vi "Save Model Digest.vi"(6 "Model group name":string="Summary", 7 "Group name":string="Summary", 8 "error in (no error)":errorcluster, 9 "Input onfiguration":T1={"Input File Path"=path "", "from scan..."=0, "...to scan"=0, "Lead resistance"=0.0, "Correct conductance "=FALSE, "Model parameters gap 1"={"Delta 1"=0.0, "Delta 2"=0.0, "Gama"=0.0, "Z"=0.0, "P"=0.0, "T"=0.0, "Integration range"=0.0, "Resolution"=0.0}, "Scale"=0.0, "Offset"=0.0, "Append channels"=[], "Model parameters gap 2"={"Delta 1"=0.0, "Delta 2"=0.0, "Gama"=0.0, "Z"=0.0, "P"=0.0, "T"=0.0, "Integration range"=0.0, "Resolution"=0.0}, "Gap 2 weight"=0.0, "Background conductance"=0.0, "Channels"=["V", "I", "dIdV"], "Preserve model history"=FALSE, "dIdV units"=enum."S"} {"Background conductance" step=0.0001 format="%#_6pS"; "Model parameters gap 2"."Delta 1" step=0.001 format="%#_6peV"; "Model parameters gap 2"."Resolution" format="%#_6peV"; "Model parameters gap 2"."Integration range" format="%#_6peV"; "Model parameters gap 2"."T" format="%#_6pK"; "Model parameters gap 2"."Delta 2" step=0.001 format="%#_6peV"; "Model parameters gap 2"."Gama" step=0.001 format="%#_6peV"; "Offset" scale=0.0..0.1; "Scale" scale=0.0..0.03; "Model parameters gap 1"."Delta 1" step=0.001 format="%#_6peV"; "Model parameters gap 1"."Resolution" format="%#_6peV"; "Model parameters gap 1"."Integration range" format="%#_6peV"; "Model parameters gap 1"."T" format="%#_6pK"; "Model parameters gap 1"."Delta 2" step=0.001 format="%#_6peV"; "Model parameters gap 1"."Gama" step=0.001 format="%#_6peV"; "Lead resistance" scale=0.0..80.0}, 11 "tdms file":refnum<k34>) -> (0 "error out":errorcluster, 1 "output group":string, 3 "tdms file out":refnum<k34>)   [LabVIEW 2021]
uses:
  Controls/PCS Config.ctl
  Parameters.ctl
panel:
  # "V"
  # "I"
  # "dIdV"
  # "<="
  # "<="
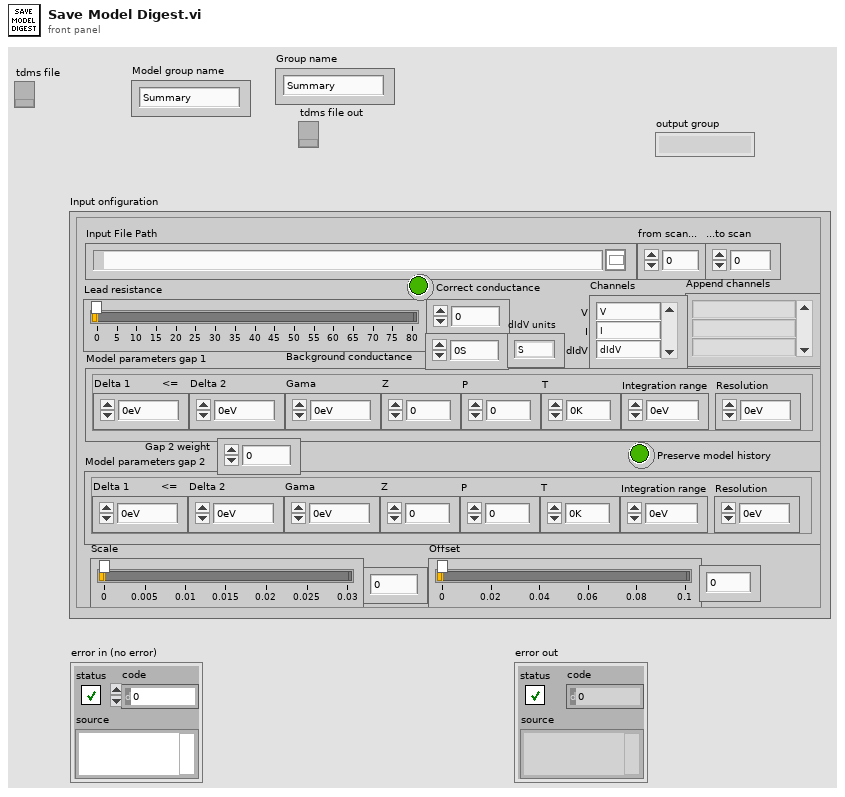
[diagram p1: front panel]
types:
  T1 = typedef "PCS Config.ctl" = cluster{"Input File Path":path, "from scan...":i32, "...to scan":i32, "Lead resistance":dbl, "Correct conductance ":bool, "Model parameters gap 1":T2, "Scale":dbl, "Offset":dbl, "Append channels":string[], "Model parameters gap 2":T2, "Gap 2 weight":dbl, "Background conductance":dbl, "Channels":string[], "Preserve model history":bool, "dIdV units":enum16{"S", "Ohm", "V"}}
  T2 = typedef "Parameters.ctl" = cluster{"Delta 1":dbl, "Delta 2":dbl, "Gama":dbl, "Z":dbl, "P":dbl, "T":dbl, "Integration range":dbl, "Resolution":dbl}
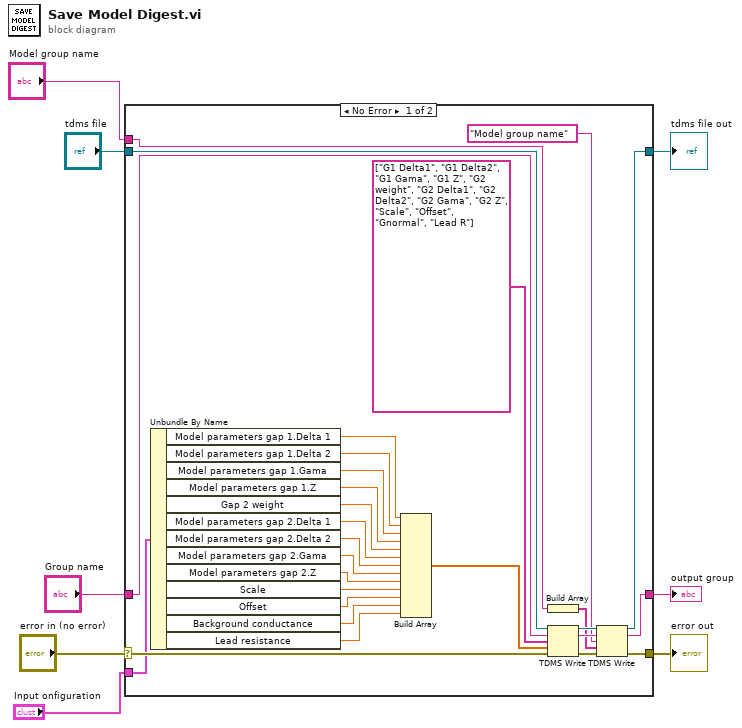
[diagram p0: block diagram]
diagram:
  n1 = case shown="No Error" "error in (no error)" {
    selector: "error in (no error)" -> [w30 w39]
    tunnel: [w31 w39] -> w7
    tunnel: "Input onfiguration" -> [w27 _]
    tunnel: [w32 w37] -> w5
    tunnel: "Group name" -> [w29 w37]
    tunnel: "tdms file" -> [w28 w38]
    tunnel: "Model group name" -> [w11 _]
    tunnel: [w9 w38] -> w1
    frame No Error {
      n2 = Unbundle By Name(w27) -> ("Model parameters gap 1.Delta 1"=w26:dbl, "Model parameters gap 1.Delta 2"=w25:dbl, "Model parameters gap 1.Gama"=w24:dbl, "Model parameters gap 1.Z"=w23:dbl, "Gap 2 weight"=w22:dbl, "Model parameters gap 2.Delta 1"=w21:dbl, "Model parameters gap 2.Delta 2"=w20:dbl, "Model parameters gap 2.Gama"=w19:dbl, "Model parameters gap 2.Z"=w18:dbl, "Scale"=w17:dbl, "Offset"=w16:dbl, "Background conductance"=w15:dbl, "Lead resistance"=w14:dbl)
      n3 = Build Array(w26, w25, w24, w23, w22, w21, w20, w19, w18, w17, w16, w15, w14) -> (w12:dbl[])
      n4 = Build Array(w11) -> (w10:string[])
      n5 = TDMS Write(0:w28, 5:w29, 7:string[] ["G1 Delta1", "G1 Delta2", "G1 Gama", "G1 Z", "G2 weight", "G2 Delta1", "G2 Delta2", "G2 Gama", "G2 Z", "Scale", "Offset", "Gnormal", "Lead R"], 9:w12, 11:w30) -> (4:w35:refnum<k34>, 6:w36:string, 15:w33:errorcluster)  [unwired: 1 in, 1 out]
      n6 = TDMS Write(0:w35, 5:w36, 7:"Model group name", 9:w10, 11:w33) -> (4:w9:refnum<k34>, 6:w32:string, 15:w31:errorcluster)  [unwired: 1 in, 1 out]
    }
    frame Error {
    }
  }
  "error out" <- w7
  "output group" <- w5
  "tdms file out" <- w1
